vi "FilepathTest.vi"() -> ()   [LabVIEW 2016]
panel:
  in  "SysDef":path
  in  "Error (in)":errorcluster
  in  "Stop Button":bool
  out "Error (out)":errorcluster
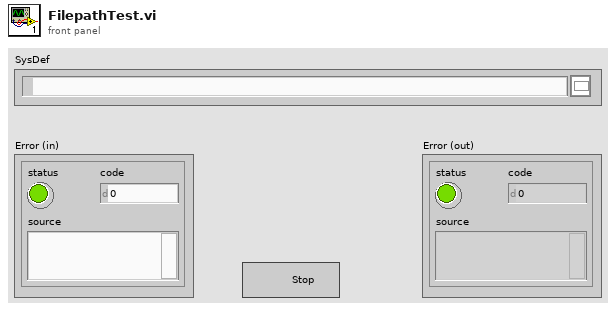
[diagram p1: front panel]
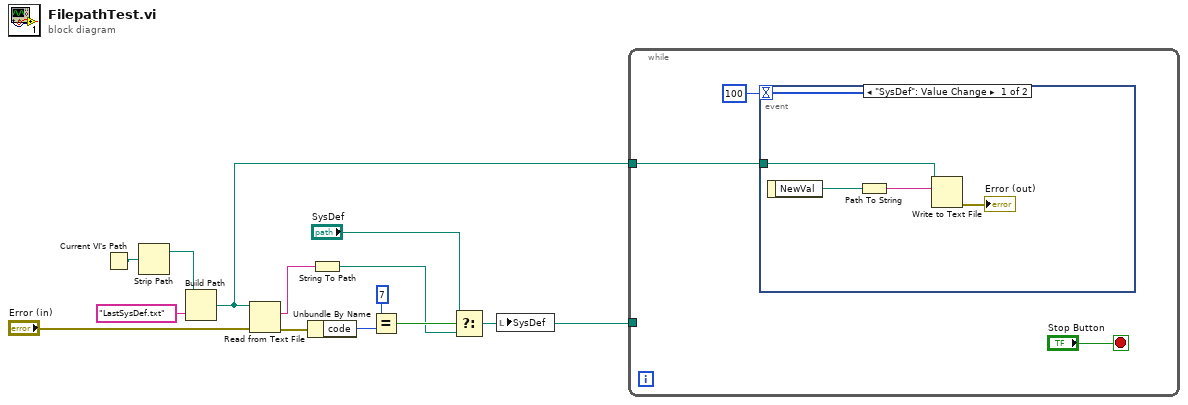
[diagram p0: block diagram]
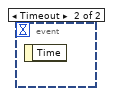
[diagram p2: hidden frame]
diagram:
  n1 = Current VI's Path() -> (path=w12:path)
  n2 = Strip Path(path=w12) -> (stripped path=w11:path)  [unwired: 1 out]
  n3 = Build Path(base path=w11, name or relative path="LastSysDef.txt") -> (appended path=w3:path)
  n4 = Read from Text File(file (use dialog)=w3, error in="Error (in)") -> (text=w6:string, error out=w10:errorcluster)  [unwired: 2 in, 2 out]
  n5 = Unbundle By Name(w10) -> ("code"=w9:i32)
  n6 = String To Path(string=w6) -> (path=w5:path)
  n7 = Equal?(x=7, y=w9) -> (x = y?=w7:bool)
  n8 = Select(t="SysDef", s=w7, f=w5) -> (s? t:f=w4:path)
  n9 = local write "SysDef"(w4) -> ()
  n10 = while {
    tunnel: w4 -> [_]
    tunnel: w3 -> [w16]
    stop <- "Stop Button" stop-if-true
    n11 = event shown="[0] \"SysDef\": Value Change" {
      selector: _ -> [_ _]
      dyn-events: _ -> [_ _]
      timeout: 100 -> [_ _]
      tunnel: w16 -> [w19 _]
      event "SysDef": Value Change {
        n12 = event-data() -> ("NewVal"=w17:path)  [unwired: 1 in]
        n13 = Path To String(path=w17) -> (string=w20:string)
        n14 = Write to Text File(file (use dialog)=w19, text=w20) -> (error out=→"Error (out)":errorcluster)  [unwired: 2 in, 2 out]
      }
      event Timeout {
        n15 = event-data() -> ()  [unwired: 1 in, 1 out]
      }
    }
  }
